vi "DigSeqLogic_One_Shot.vi"(8 "Time":dbl=-1.0, 9 "OneShot":dbl=1.0, 11 "Input":bool) -> (1 "Remain":dbl, 3 "Output":bool)   [LabVIEW 2019, in "Trajectory_Library.lvlib"]
doc: "This VI implements a digital \"one shot\". The output is true for a specific period of time after the input transitions from FALSE to TRUE.\n\nInputs:\n - Input -- Boolean input to use for one shot output\n - OneShot -- Length of one shot output in seconds.\n - Time -- Current system time. If not wired, FPGA time is used. \n\nOutput:\n - Output -- Boolean output one-shot \n - Remain -- Number of seconds remaining in one-shot."
uses:
  Trajectory_Library.lvlib
  <vilib>/Utility/semaphor.llb/Obtain Semaphore Reference.vi
  Timer_Reset.vi
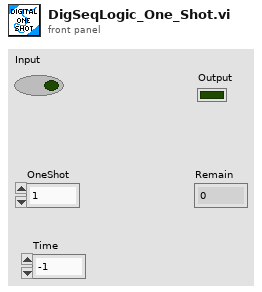
[diagram p1: front panel]
types:
  T1 = typedef "Trajectory_Library.lvlib/TIMER.ctl" = cluster{"StartTime":dbl, "Accumulated TIme":dbl, "Running":bool, "semaphore":T2}
  T2 = typedef "Semaphore RefNum" = refnum<k1>
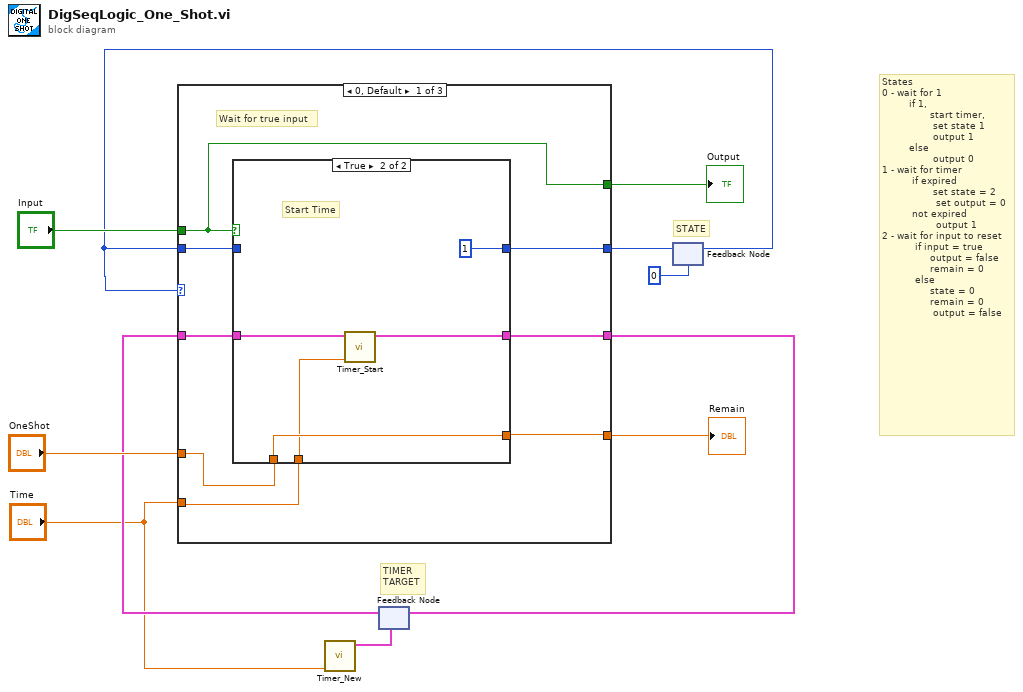
[diagram p0: block diagram]
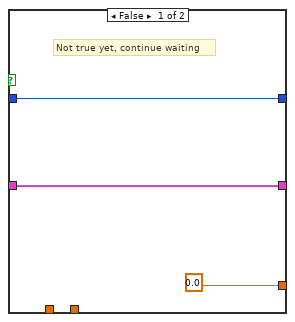
[diagram p2: hidden frame]
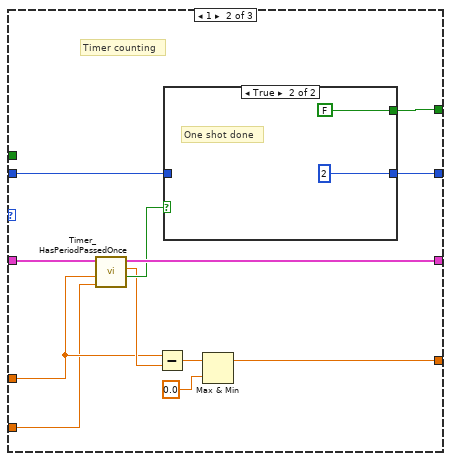
[diagram p3: hidden frame]
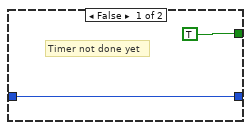
[diagram p4: hidden frame]
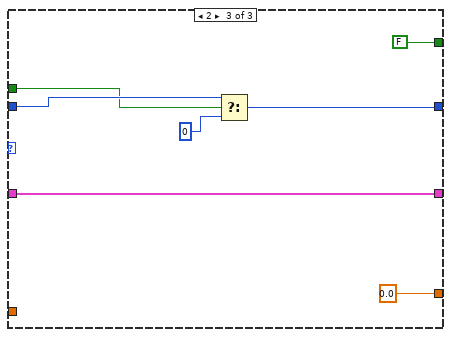
[diagram p5: hidden frame]
diagram:
  # "TIMER\nTARGET"
  # "STATE"
  # "States \n0 - wait for 1\n         if 1, \n                start timer, \n                 set state 1\n                 output 1\n         else\n                 output 0\n1 - wait for timer\n          if expired\n                 set state = 2\n                  set output = 0 \n          not expired\n                  output 1\n2 - wait for input to reset\n           if input = true\n                output = false\n                remain = 0\n           else\n                state = 0\n                remain = 0\n                 output = false"
  n1 = call "Timer_New.vi"("Pass_Through_Time"="Time") -> ("TIMER"=w4:T1)  [unwired: 10 in]
  n2 = feedback #1(w4) -> (w3:T1)
  n3 = feedback #2(0 ("State")) -> (w6:i32)
  n4 = case shown="0, Default" w6 {
    tunnel: "OneShot" -> [w17 w30 _]
    tunnel: "Time" -> [w19 w28 _]
    tunnel: [w16 w39 FALSE ("Output")] -> w10
    tunnel: [w18 w29 0.0 ("Remain")] -> w9
    tunnel: "Input" -> [w16 _ w45]
    tunnel: [w15 w38 w44] -> w7
    tunnel: w6 -> [w14 w37 w47]
    tunnel: [w13 w35 w48] -> w2
    tunnel: w3 -> [w12 w36 w48]
    frame 0, Default {
      # "Wait for true input"
      n5 = case shown="True" w16 {
        tunnel: w17 -> [_ w27]
        tunnel: w19 -> [_ w23]
        tunnel: [0.0 ("OneShot") w27] -> w18
        tunnel: [w21 1 ("State")] -> w15
        tunnel: w14 -> [w21 _]
        tunnel: [w20 w25] -> w13
        tunnel: w12 -> [w20 w24]
        frame False {
          # "Not true yet, continue waiting"
        }
        frame True {
          # "Start Time"
          n6 = call "Timer_Start.vi"("Pass_Through_Time"=w23, "in Timer"=w24) -> ("out Timer"=w25:T1)  [unwired: 9 in]
        }
      }
    }
    frame 1 {
      # "Timer counting"
      n7 = call "Timer_HasPeriodPassedOnce.vi"("Pass_Through_Time"=w28, "Period"=w30, "in Timer"=w36) -> ("Expired"=w34:bool, "CurrentTImer"=w31:dbl, "out Timer"=w35:T1)  [unwired: 6 in]
      n8 = Subtract(x=w30, y=w31) -> (x-y=w32:dbl)
      n9 = case shown="True" w34 {
        tunnel: [TRUE FALSE] -> w39
        tunnel: [w40 2 ("State")] -> w38
        tunnel: w37 -> [w40 _]
        frame False {
          # "Timer not done yet"
        }
        frame True {
          # "One shot done"
        }
      }
      n10 = Max & Min(x=w32, y=0.0) -> (max(x,y)=w29:dbl)  [unwired: 1 out]
    }
    frame 2 {
      n11 = Select(t=w47, s=w45, f=0 ("State")) -> (s? t:f=w44:i32)
    }
  }
  "Remain" <- w9
  "Output" <- w10
  n12 = feedback-in #1(w2) -> ()
  n13 = feedback-in #2(w7) -> ()
